vi "IOtest.vi"   [LabVIEW 2014]
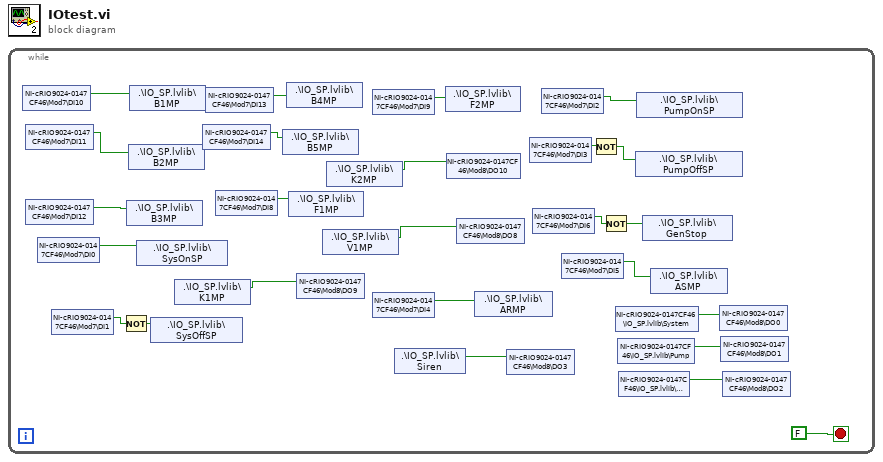
[diagram p0: block diagram]
diagram:
  n1 = while {
    stop <- FALSE stop-if-true
    n2 = shared-variable "NI-cRIO9024-0147CF46\\Mod7\\DI10"() -> (w25:bool)  [unwired: 1 in, 1 out]
    n3 = shared-variable "NI-cRIO9024-0147CF46\\Mod7\\DI11"() -> (w24:bool)  [unwired: 1 in, 1 out]
    n4 = shared-variable "NI-cRIO9024-0147CF46\\Mod7\\DI12"() -> (w23:bool)  [unwired: 1 in, 1 out]
    n5 = shared-variable "NI-cRIO9024-0147CF46\\Mod7\\DI0"() -> (w20:bool)  [unwired: 1 in, 1 out]
    n6 = shared-variable "NI-cRIO9024-0147CF46\\Mod7\\DI1"() -> (w5:bool)  [unwired: 1 in, 1 out]
    n7 = Not(x=w5) -> (.not. x?=w4:bool)
    n8 = shared-variable ".\\IO_SP.lvlib\\B3MP"(w23) -> ()  [unwired: 1 in, 1 out]
    n9 = shared-variable ".\\IO_SP.lvlib\\B2MP"(w24) -> ()  [unwired: 1 in, 1 out]
    n10 = shared-variable ".\\IO_SP.lvlib\\B1MP"(w25) -> ()  [unwired: 1 in, 1 out]
    n11 = shared-variable ".\\IO_SP.lvlib\\SysOnSP"(w20) -> ()  [unwired: 1 in, 1 out]
    n12 = shared-variable ".\\IO_SP.lvlib\\SysOffSP"(w4) -> ()  [unwired: 1 in, 1 out]
    n13 = shared-variable ".\\IO_SP.lvlib\\K1MP"() -> (w12:bool)  [unwired: 1 in, 1 out]
    n14 = shared-variable "NI-cRIO9024-0147CF46\\Mod7\\DI14"() -> (w21:bool)  [unwired: 1 in, 1 out]
    n15 = shared-variable "NI-cRIO9024-0147CF46\\Mod7\\DI13"() -> (w22:bool)  [unwired: 1 in, 1 out]
    n16 = shared-variable "NI-cRIO9024-0147CF46\\Mod7\\DI8"() -> (w16:bool)  [unwired: 1 in, 1 out]
    n17 = shared-variable ".\\IO_SP.lvlib\\B5MP"(w21) -> ()  [unwired: 1 in, 1 out]
    n18 = shared-variable ".\\IO_SP.lvlib\\B4MP"(w22) -> ()  [unwired: 1 in, 1 out]
    n19 = shared-variable ".\\IO_SP.lvlib\\F1MP"(w16) -> ()  [unwired: 1 in, 1 out]
    n20 = shared-variable "NI-cRIO9024-0147CF46\\Mod8\\DO9"(w12) -> ()  [unwired: 1 in, 1 out]
    n21 = shared-variable ".\\IO_SP.lvlib\\V1MP"() -> (w11:bool)  [unwired: 1 in, 1 out]
    n22 = shared-variable ".\\IO_SP.lvlib\\K2MP"() -> (w13:bool)  [unwired: 1 in, 1 out]
    n23 = shared-variable "NI-cRIO9024-0147CF46\\Mod7\\DI9"() -> (w15:bool)  [unwired: 1 in, 1 out]
    n24 = shared-variable "NI-cRIO9024-0147CF46\\Mod7\\DI4"() -> (w19:bool)  [unwired: 1 in, 1 out]
    n25 = shared-variable ".\\IO_SP.lvlib\\Siren"() -> (w14:bool)  [unwired: 1 in, 1 out]
    n26 = shared-variable ".\\IO_SP.lvlib\\F2MP"(w15) -> ()  [unwired: 1 in, 1 out]
    n27 = shared-variable "NI-cRIO9024-0147CF46\\Mod8\\DO10"(w13) -> ()  [unwired: 1 in, 1 out]
    n28 = shared-variable "NI-cRIO9024-0147CF46\\Mod8\\DO8"(w11) -> ()  [unwired: 1 in, 1 out]
    n29 = shared-variable ".\\IO_SP.lvlib\\ARMP"(w19) -> ()  [unwired: 1 in, 1 out]
    n30 = shared-variable "NI-cRIO9024-0147CF46\\Mod8\\DO3"(w14) -> ()  [unwired: 1 in, 1 out]
    n31 = shared-variable "NI-cRIO9024-0147CF46\\Mod7\\DI3"() -> (w7:bool)  [unwired: 1 in, 1 out]
    n32 = shared-variable "NI-cRIO9024-0147CF46\\Mod7\\DI6"() -> (w8:bool)  [unwired: 1 in, 1 out]
    n33 = shared-variable "NI-cRIO9024-0147CF46\\Mod7\\DI2"() -> (w10:bool)  [unwired: 1 in, 1 out]
    n34 = shared-variable "NI-cRIO9024-0147CF46\\Mod7\\DI5"() -> (w18:bool)  [unwired: 1 in, 1 out]
    n35 = Not(x=w7) -> (.not. x?=w6:bool)
    n36 = Not(x=w8) -> (.not. x?=w9:bool)
    n37 = shared-variable "NI-cRIO9024-0147CF46\\IO_SP.lvlib\\System"() -> (w3:bool)  [unwired: 1 in, 1 out]
    n38 = shared-variable "NI-cRIO9024-0147CF46\\IO_SP.lvlib\\Pump"() -> (w2:bool)  [unwired: 1 in, 1 out]
    n39 = shared-variable "NI-cRIO9024-0147CF46\\IO_SP.lvlib\\Fault"() -> (w1:bool)  [unwired: 1 in, 1 out]
    n40 = shared-variable ".\\IO_SP.lvlib\\PumpOffSP"(w6) -> ()  [unwired: 1 in, 1 out]
    n41 = shared-variable ".\\IO_SP.lvlib\\PumpOnSP"(w10) -> ()  [unwired: 1 in, 1 out]
    n42 = shared-variable ".\\IO_SP.lvlib\\GenStop"(w9) -> ()  [unwired: 1 in, 1 out]
    n43 = shared-variable ".\\IO_SP.lvlib\\ASMP"(w18) -> ()  [unwired: 1 in, 1 out]
    n44 = shared-variable "NI-cRIO9024-0147CF46\\Mod8\\DO0"(w3) -> ()  [unwired: 1 in, 1 out]
    n45 = shared-variable "NI-cRIO9024-0147CF46\\Mod8\\DO1"(w2) -> ()  [unwired: 1 in, 1 out]
    n46 = shared-variable "NI-cRIO9024-0147CF46\\Mod8\\DO2"(w1) -> ()  [unwired: 1 in, 1 out]
  }
